vi "Index Arrays - I32.vi"(9 "Index array":u32[](array[numeric]), 11 "Array in":i32[](array[numeric])) -> (3 "Array out":i32[](array[numeric]))   [LabVIEW 2014]
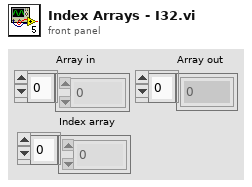
[diagram p1: front panel]
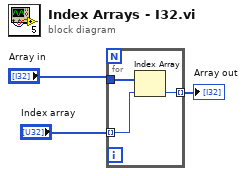
[diagram p0: block diagram]
diagram:
  n1 = for {
    tunnel: "Array in" -> [w6]
    tunnel: "Index array" -> [w5] mode=indexing
    tunnel: [w4] -> w1 mode=indexing
    n2 = Index Array(array=w6, index=w5) -> (element=w4:i32)
  }
  "Array out" <- w1
